vi "Kinect Acquire From File.vi"(8 "error in":errorcluster, 11 "Path to Folder\nContaining TIFF Images":path=path "C:/Users/Behavior Room/Desktop/Recordings/Single Mouse") -> (0 "error out":errorcluster, 1 "Out of Frames?":bool, 2 "Diff Image Out":T1(plugin-control), 3 "Image Out":T1(plugin-control))   [LabVIEW 2011]
uses:
  <vilib>/vision/NI_Vision_Development_Module.lvlib
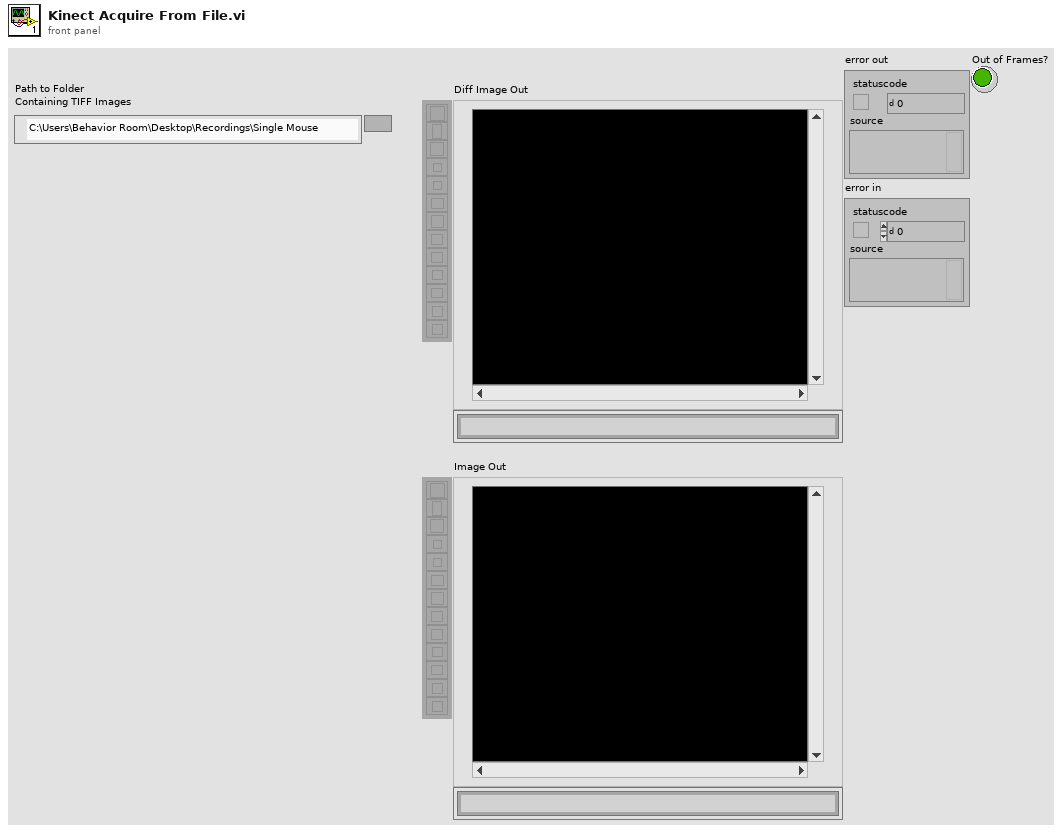
[diagram p1: front panel]
types:
  T1 = typedef "IMAQ Image.ctl" = refnum<image>
  T2 = typedef "Image Type" = u32
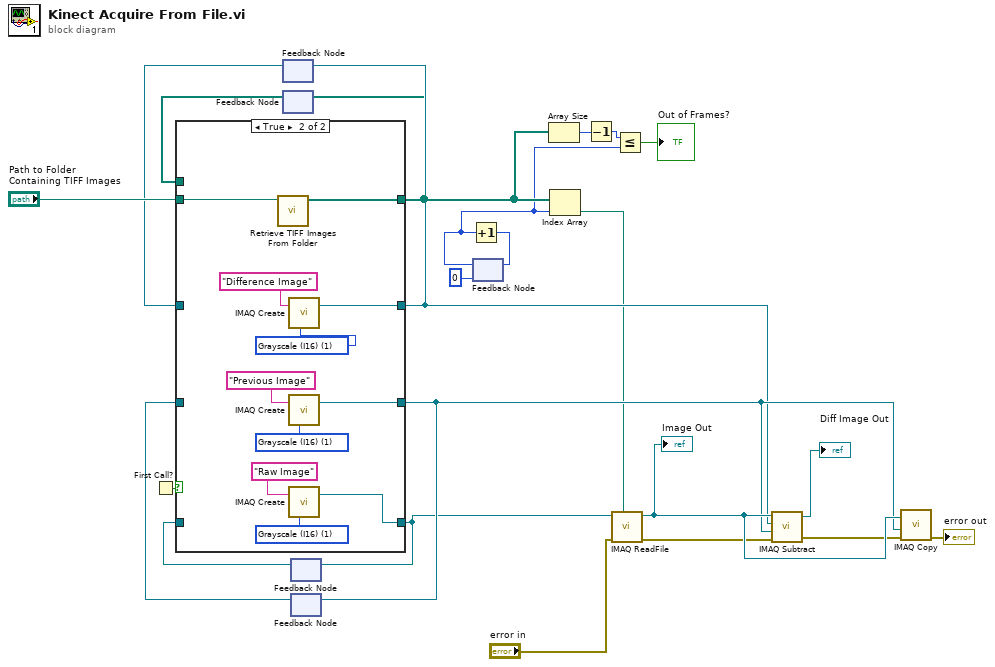
[diagram p0: block diagram]
diagram:
  n1 = First Call?() -> (First Call?: T/F=w14:bool)
  n2 = feedback #1() -> (w12:T1)  [unwired: 1 in]
  n3 = feedback #2() -> (w15:path[])  [unwired: 1 in]
  n4 = feedback #3() -> (w13:T1)  [unwired: 1 in]
  n5 = feedback #4() -> (w11:T1)  [unwired: 1 in]
  n6 = case shown="True" w14 {
    tunnel: [w27 w36] -> w17
    tunnel: w13 -> [w27 _]
    tunnel: [w26 w34] -> w20
    tunnel: w12 -> [w26 _]
    tunnel: [w25 w30] -> w22
    tunnel: w11 -> [w25 _]
    tunnel: [w24 w29] -> w5
    tunnel: w15 -> [w24 _]
    tunnel: "Path to Folder\nContaining TIFF Images" -> [_ w28]
    frame False {
    }
    frame True {
      w32 = T2 1 items=["Grayscale (U8)", "Grayscale (I16)", "Grayscale (SGL)", "Complex (CSG)", "RGB (U32)", "HSL (U32)", "RGB (U64)", "Grayscale (U16)"] ("Image Type")
      w33 = T2 1 items=["Grayscale (U8)", "Grayscale (I16)", "Grayscale (SGL)", "Complex (CSG)", "RGB (U32)", "HSL (U32)", "RGB (U64)", "Grayscale (U16)"] ("Image Type")
      w37 = T2 1 items=["Grayscale (U8)", "Grayscale (I16)", "Grayscale (SGL)", "Complex (CSG)", "RGB (U32)", "HSL (U32)", "RGB (U64)", "Grayscale (U16)"] ("Image Type")
      n7 = call "Retrieve TIFF Images From Folder.vi"("Path to Folder\nContaining TIFF Images"=w28) -> ("Array of TIFF Image Paths"=w29:path[])  [unwired: 10 in]
      n8 = call "IMAQ Create"("Image Name"="Difference Image", "Image Type"=w33) -> ("New Image"=w34:T1)  [unwired: 3 in, 1 out]
      n9 = call "IMAQ Create"("Image Name"="Previous Image", "Image Type"=w32) -> ("New Image"=w30:T1)  [unwired: 3 in, 1 out]
      n10 = call "IMAQ Create"("Image Name"="Raw Image", "Image Type"=w37) -> ("New Image"=w36:T1)  [unwired: 3 in, 1 out]
    }
  }
  n11 = feedback-in #1(w20) -> ()
  n12 = feedback-in #2(w5) -> ()
  n13 = feedback-in #3(w17) -> ()
  n14 = feedback-in #4(w22) -> ()
  n15 = feedback #5(0) -> (w4:i32)
  n16 = Increment(x=w4) -> (x+1=w10:i32)
  n17 = feedback-in #5(w10) -> ()
  n18 = Array Size(array=w5) -> (size(s)=w2:i32)
  n19 = Index Array(array=w5, index=w4) -> (element=w8:path)
  n20 = Decrement(x=w2) -> (x-1=w1:i32)
  n21 = call "IMAQ ReadFile"("File Path"=w8, "error in (no error)"="error in", "Image"=w17) -> ("error out"=w21:errorcluster, "Image Out"=w23:T1)  [unwired: 4 in, 3 out]
  "Image Out" <- w23
  n22 = Less Or Equal?(x=w1, y=w4) -> (x <= y?=→"Out of Frames?":bool)
  n23 = call "IMAQ Subtract"("Image Src A"=w23, "Image Dst"=w20, "Image Src B"=w22, "error in (no error)"=w21) -> ("Image Dst Out"=→"Diff Image Out":T1, "error out"=w19:errorcluster)  [unwired: 3 in]
  n24 = call "IMAQ Copy"("error in (no error)"=w19, "Image Dst"=w22, "Image Src"=w23) -> ("error out"=→"error out":errorcluster)  [unwired: 3 in, 1 out]
